vi "Write Image Prefix.vi"(8 "error in (no error)":errorcluster, 10 "Prefix":string, 11 "HIJ IMAQdx Camera Viewer in":refnum<class "HIJ IMAQdx Camera Viewer.lvclass">) -> (0 "error out":errorcluster, 3 "HIJ IMAQdx Camera Viewer out":refnum<class "HIJ IMAQdx Camera Viewer.lvclass">)   [LabVIEW 2014, in "HIJ IMAQdx Justage Camera w Timer.lvlib" / "HIJ IMAQdx Camera Viewer.lvclass"]
uses:
  HIJ IMAQdx Camera Viewer.lvclass
  HIJ IMAQdx Camera Viewer.lvclass/HIJ IMAQdx Camera Viewer.ctl
  Applications/HIJ Vision Camera App/HIJ Vision Camera App/HIJ Vision Camera App.lvclass
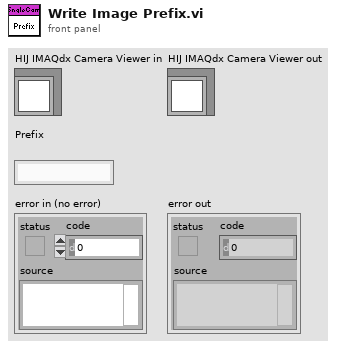
[diagram p1: front panel]
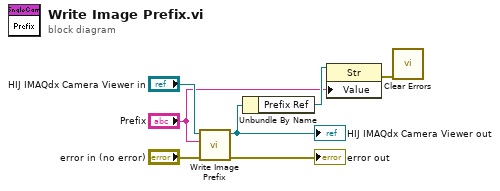
[diagram p0: block diagram]
diagram:
  n1 = call-parent "Write Image Prefix.vi"("error in (no error)"="error in (no error)", "Prefix"="Prefix", "HIJ Vision Application in"="HIJ IMAQdx Camera Viewer in") -> ("error out"=→"error out":errorcluster, "HIJ Vision Application out"=w4:refnum<class "HIJ IMAQdx Camera Viewer.lvclass">)  [unwired: 7 in]
  "HIJ IMAQdx Camera Viewer out" <- w4
  n2 = Unbundle By Name(w4) -> ("Prefix Ref"=w3:refnum<vi>)
  n3 = property class="Str"(reference=w3, "Value"="Prefix") -> (error out=w1:errorcluster)  [unwired: 1 in, 1 out]
  n4 = call <vilib>:"Clear Errors.vi"("error in (no error)"=w1) -> ()  [unwired: 5 in, 2 out]
